vi "Untitled 2.vi"() -> ()   [LabVIEW 2019]
panel:
  in  "Ferramenta":string
  in  "Temperatura 2":dbl
  in  "Temperatura 1":dbl
  in  "Ordem de serviço":string
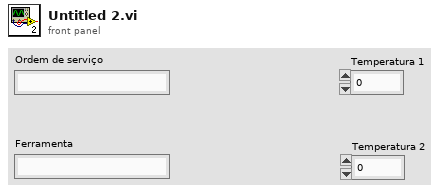
[diagram p1: front panel]
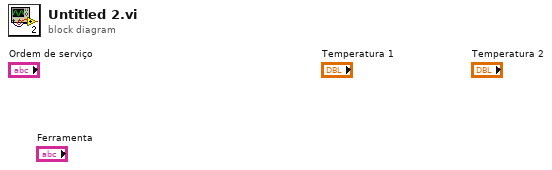
[diagram p0: block diagram]
diagram:
